vi "MD5, Calculate Message-Digest.vi"(2 "size (in bytes)":i64, 3 "data":string) -> (0 "MD5 message-digest":string)   [LabVIEW 2010]
doc: "Computes the MD5 message-digest of a buffer. The MD5 message-digest is a 128-bit number displayed in lowercase hexadecimal format."
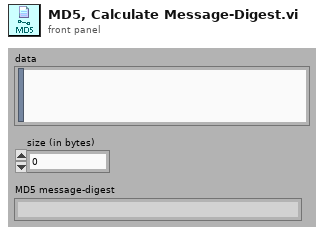
[diagram p1: front panel]
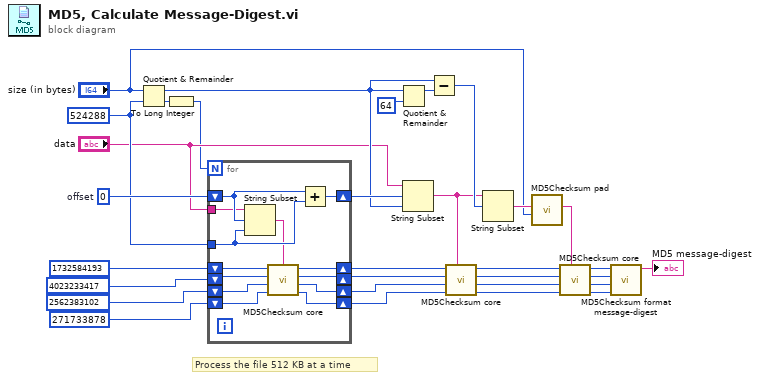
[diagram p0: block diagram]
diagram:
  w23 = i64 0  # offset
  w10 = i64 524288 ("y")
  # "Process the file 512 KB at a time"
  n1 = Quotient & Remainder(x="size (in bytes)", y=w10) -> (x-y*floor(x/y)=w7:i64, floor(x/y)=w31:i64)
  n2 = To Long Integer(number=w31) -> (32bit integer=w3:i32)
  n3 = for {
    N: w3 -> [_]
    shift-right: [w41] -> w26
    shift-left: u32 1732584193 ("s1") -> [w44]
    shift-right: [w40] -> w25
    shift-left: u32 4023233417 ("s2") -> [w43]
    shift-right: [w39] -> w1
    shift-left: u32 2562383102 ("s3") -> [w32]
    shift-right: [w38] -> w2
    shift-left: u32 271733878 ("s4") -> [w42]
    shift-right: [w37] -> w8
    shift-left: w23 -> [w34]
    tunnel: w10 -> [w36]
    tunnel: "data" -> [w33]
    n4 = String Subset(string=w33, offset (0)=w34, length (rest)=w36) -> (substring=w35:string)
    n5 = call <vilib>:"MD5Checksum core.vi"("Input String"=w35, "s4 in"=w42, "s3 in"=w32, "s2 in"=w43, "s1 in"=w44) -> ("s4 out"=w38:u32, "s3 out"=w39:u32, "s2 out"=w40:u32, "s1 out"=w41:u32)  [unwired: 3 in]
    n6 = Add(x=w34, y=w36) -> (x+y=w37:i64)
  }
  n7 = Quotient & Remainder(x=w7, y=i64 64) -> (x-y*floor(x/y)=w22:i64)  [unwired: 1 out]
  n8 = String Subset(string="data", offset (0)=w8, length (rest)=w7) -> (substring=w6:string)
  n9 = Subtract(x=w7, y=w22) -> (x-y=w21:i64)
  n10 = call <vilib>:"MD5Checksum core.vi"("Input String"=w6, "s4 in"=w2, "s3 in"=w1, "s2 in"=w25, "s1 in"=w26) -> ("s4 out"=w16:u32, "s3 out"=w17:u32, "s2 out"=w18:u32, "s1 out"=w19:u32)  [unwired: 3 in]
  n11 = String Subset(string=w6, offset (0)=w21) -> (substring=w20:string)  [unwired: 1 in]
  n12 = call <vilib>:"MD5Checksum pad.vi"("Message String Length (bytes)"="size (in bytes)", "Last Part of Message String"=w20) -> ("Padding"=w15:string)  [unwired: 9 in]
  n13 = call <vilib>:"MD5Checksum core.vi"("Input String"=w15, "s4 in"=w16, "s3 in"=w17, "s2 in"=w18, "s1 in"=w19) -> ("s4 out"=w11:u32, "s3 out"=w12:u32, "s2 out"=w13:u32, "s1 out"=w14:u32)  [unwired: 3 in]
  n14 = call <vilib>:"MD5Checksum format message-digest.vi"("s4"=w11, "s3"=w12, "s2"=w13, "s1"=w14) -> ("MD5 message-digest"=→"MD5 message-digest":string)  [unwired: 7 in]
